vi "IV.vi"() -> ()   [LabVIEW 2018]
uses:
  Classes/2D/IV/IV.lvclass
  Classes/2D/IV/data/IV_data.lvclass
  Classes/2D/IV/meas/IV_meas.lvclass
  support/Message Queue/Enqueue Message (Single).vi
  Classes/Abstract/Measurement/Measurement2D/Measurement2D.lvclass
  Classes/Abstract/Data/Data2D/Data2D.lvclass
  support/Message Queue/Kapitza Message Queue.lvlib
  support/User Event - Stop/Kapitza User Event - Stop.lvlib
panel:
  out "Current Step":dbl[unit]
  out "dV/dI":dbl caption="dV/dI, Ohm"
  in  "Tab Control":enum32{"IV", "dV/dI (I)"}(tab)
  out "IV":cluster{"X":dbl[], "Y":dbl[]}[](graph)
  out "dV/dI (I)":cluster{"X":dbl[], "Y":dbl[]}[](graph) caption="IV"
  in  "File Path Control":path=path "C:/Users/Sergei/Documents"
  in  "Driver 1":path=path "C:/Users/Sergei/YandexDisk/Лаборатория/Projects/Kapitza_prealpha/Drivers/Simulator.vi" caption="Current source driver"
  in  "Driver 2":path=path "C:/Users/Sergei/YandexDisk/Лаборатория/Projects/Kapitza_prealpha/Drivers/Simulator.vi" caption="Voltmeter driver"
  in  "Address 2":refnum<visa-resource-name> caption="Voltmeter"
  in  "Address 1":refnum<visa-resource-name> caption="Current source"
  in  "Stop":bool
  in  "Sample Name":string
  in  "Max":dbl caption="Max current, uA"
  in  "Step":dbl caption="Current step, uA"
  in  "Init":dbl caption="Init current, uA"
  in  "x0,5 step":bool
  out "V":dbl caption="V, uV"
  out "I":dbl caption="I, uA"
  in  "x2 step":bool
  in  "Start":bool
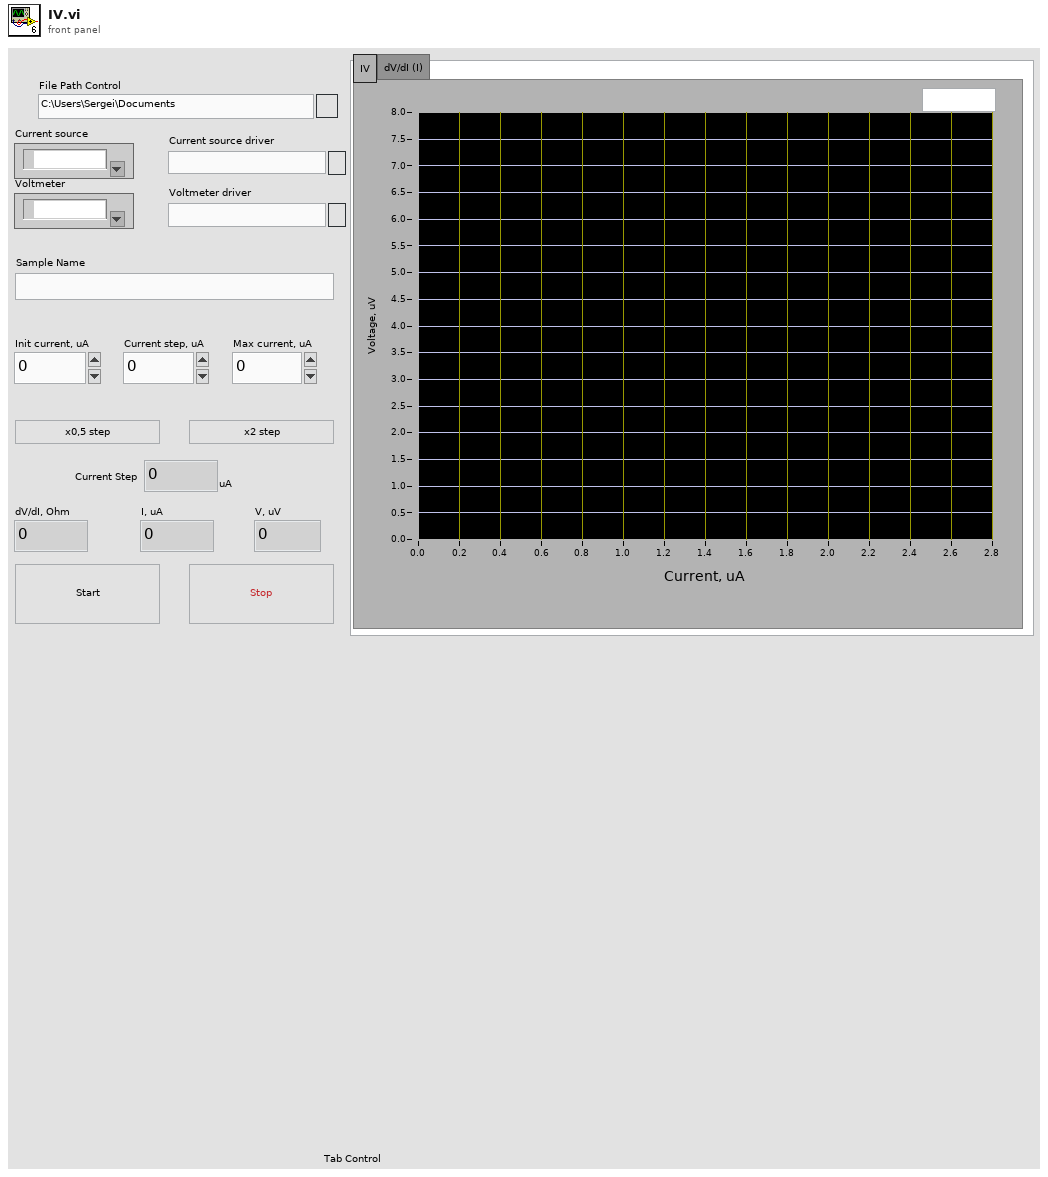
[diagram p1: front panel]
types:
  T1 = typedef "Kapitza Message Queue.lvlib/All Message Queues.ctl" = cluster{"UI":refnum<queue>}
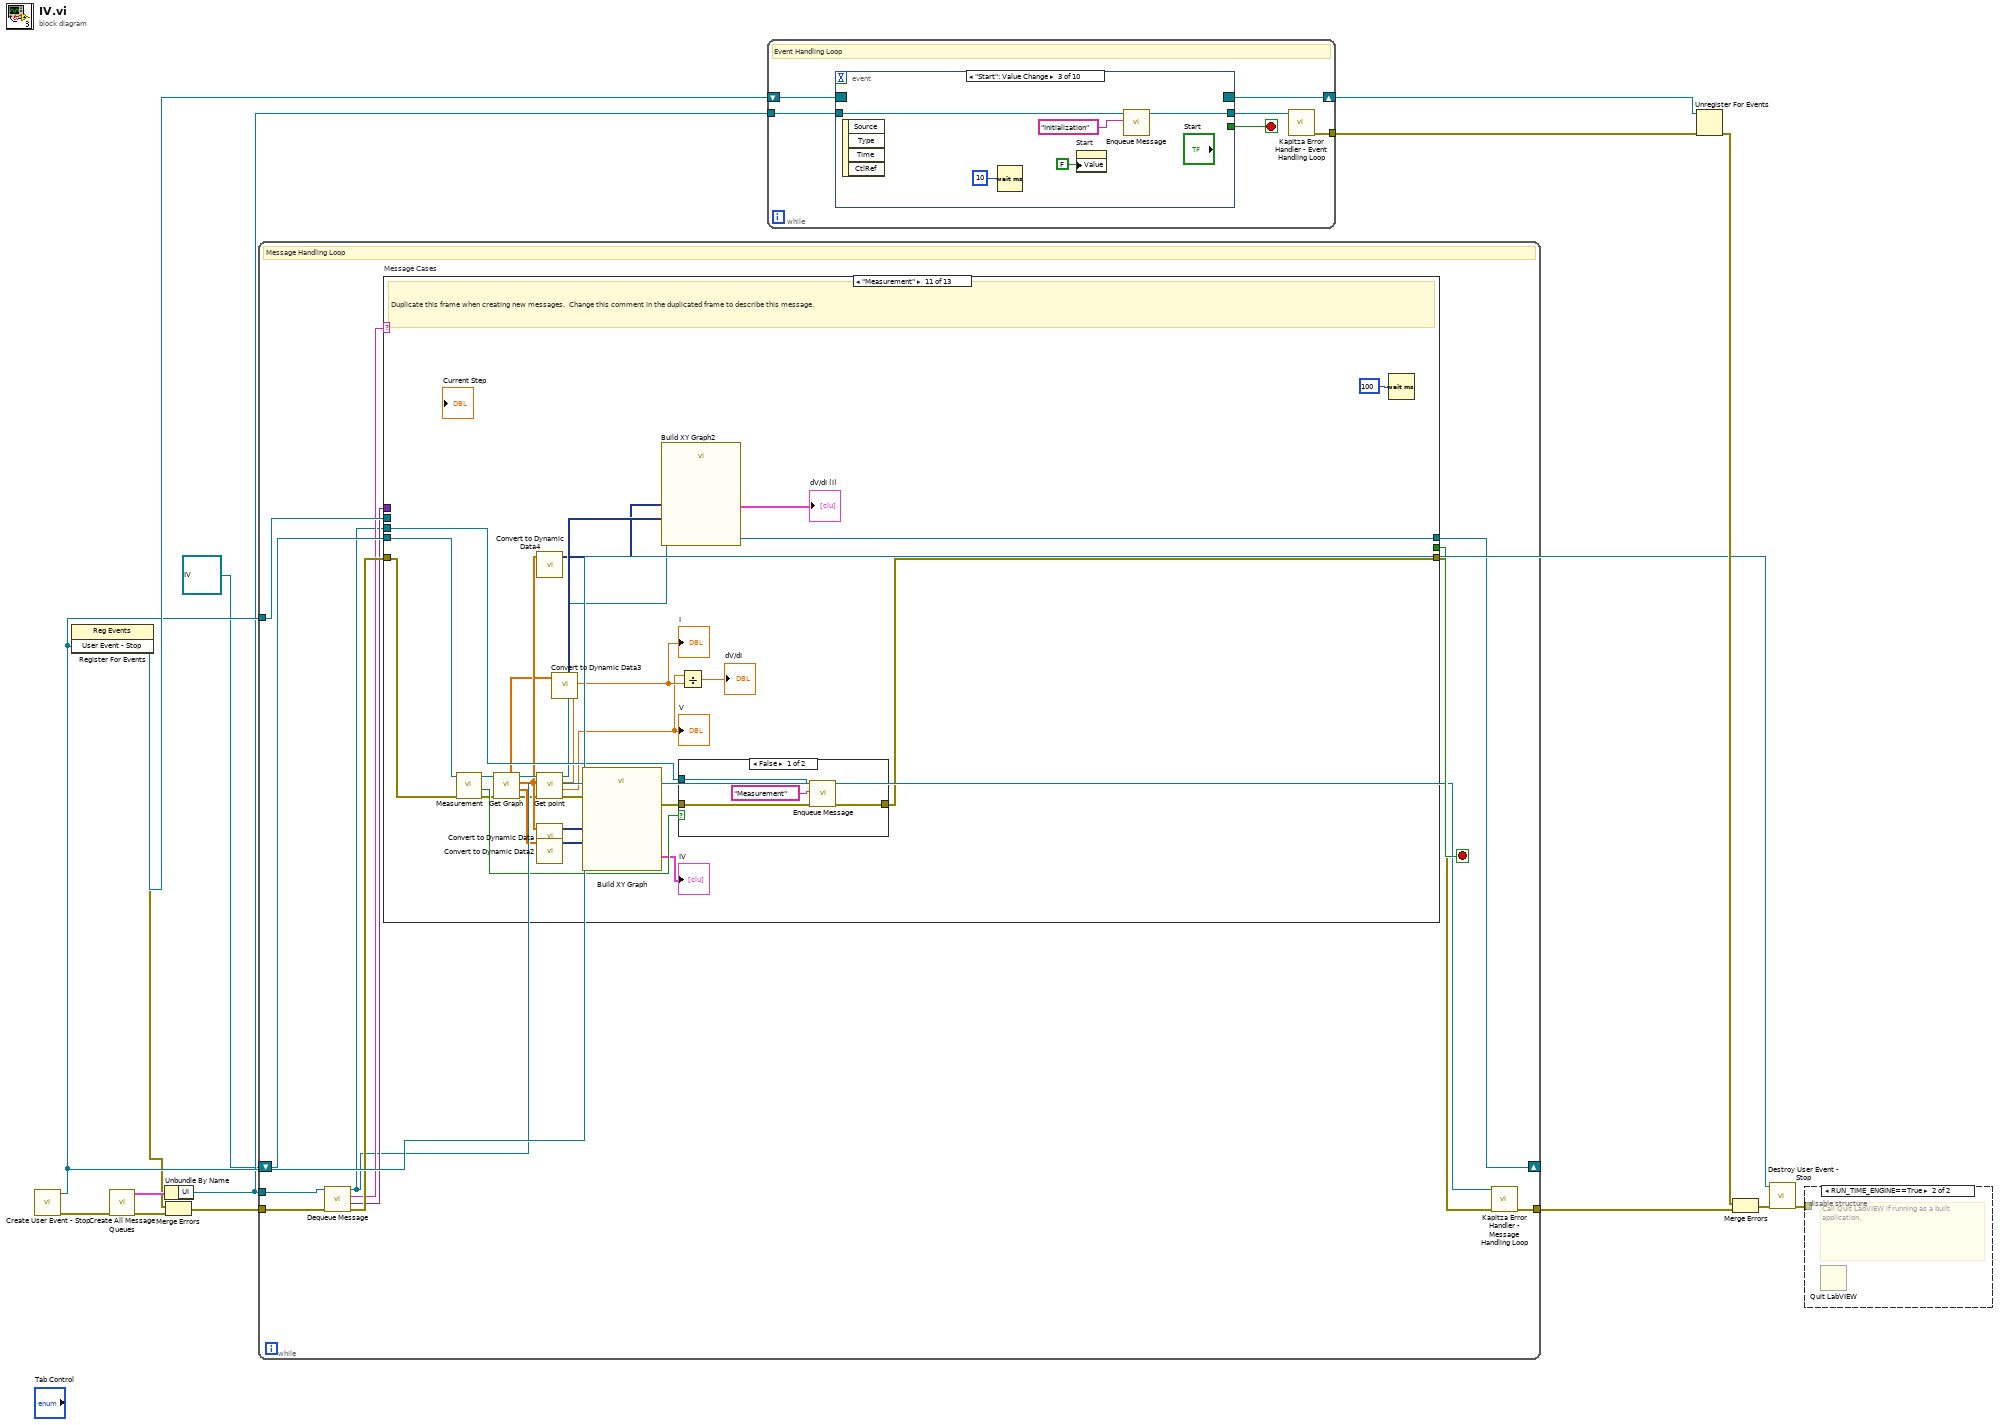
[diagram p0: block diagram]
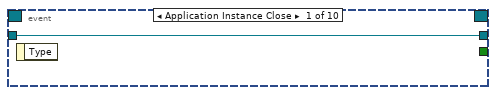
[diagram p3: hidden frame]
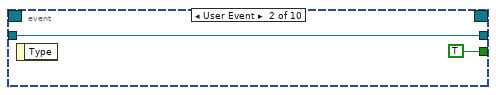
[diagram p4: hidden frame]
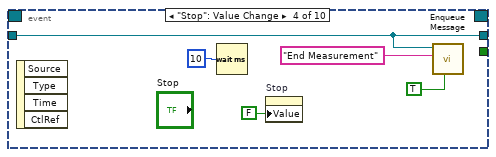
[diagram p5: hidden frame]
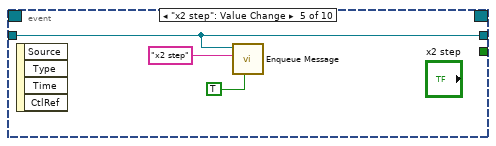
[diagram p6: hidden frame]
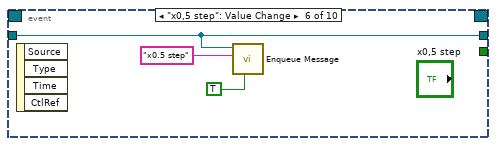
[diagram p7: hidden frame]
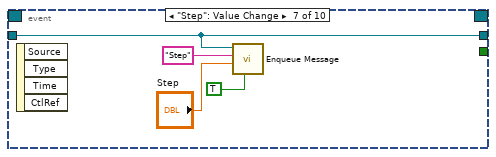
[diagram p8: hidden frame]
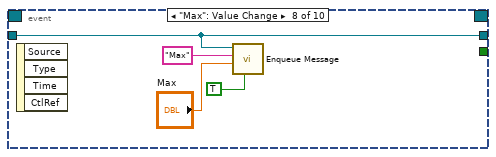
[diagram p9: hidden frame]
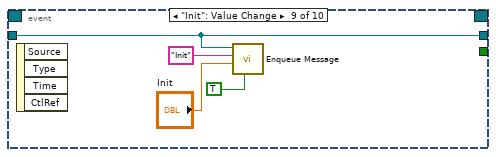
[diagram p10: hidden frame]
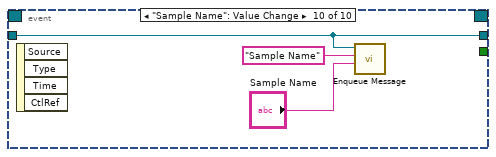
[diagram p11: hidden frame]
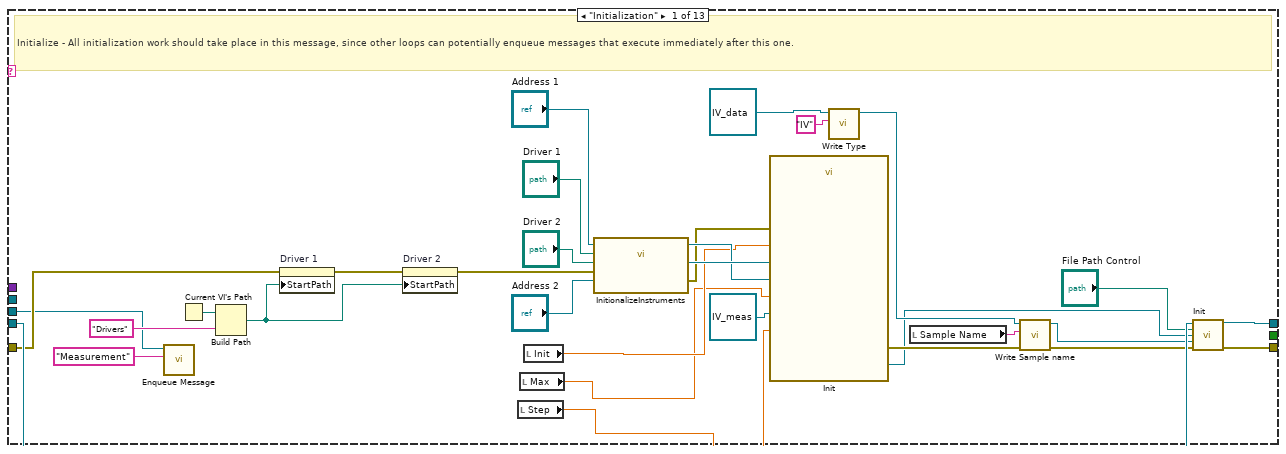
[diagram p12: hidden frame]
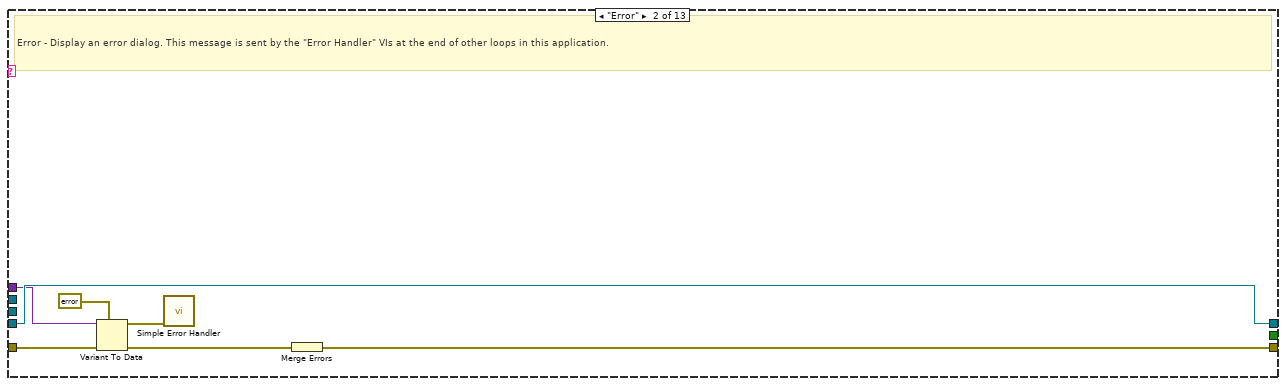
[diagram p13: hidden frame]
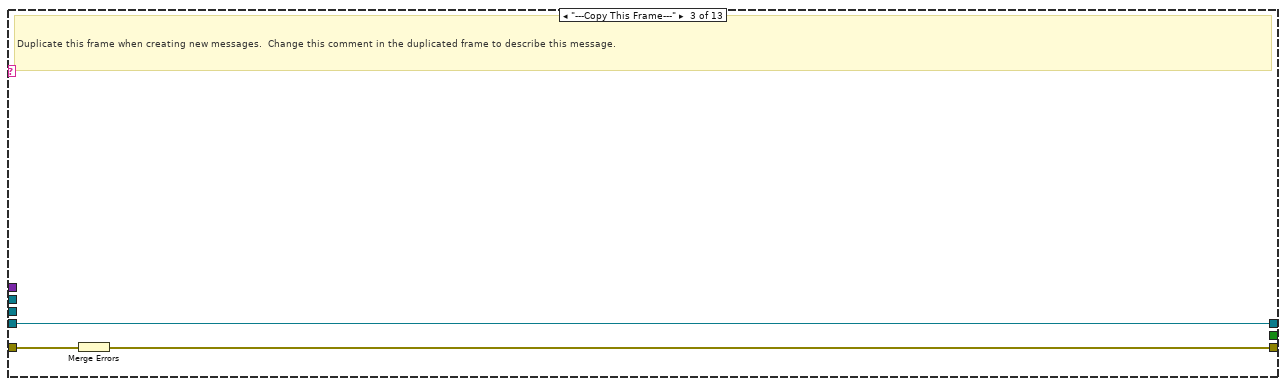
[diagram p14: hidden frame]
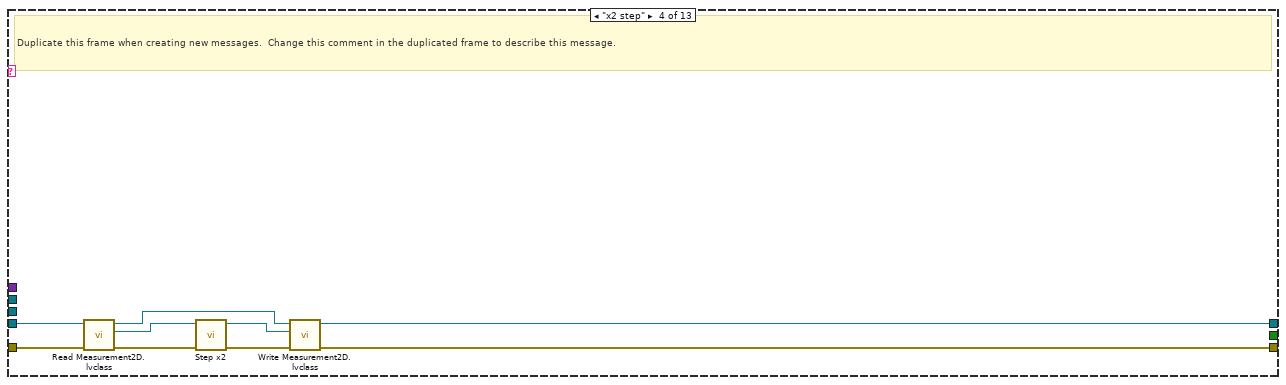
[diagram p15: hidden frame]
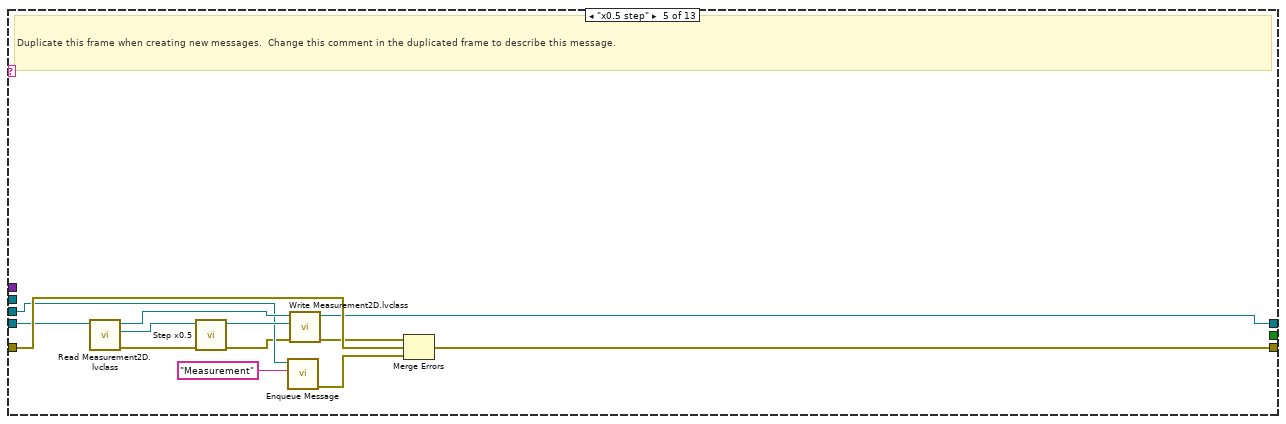
[diagram p16: hidden frame]
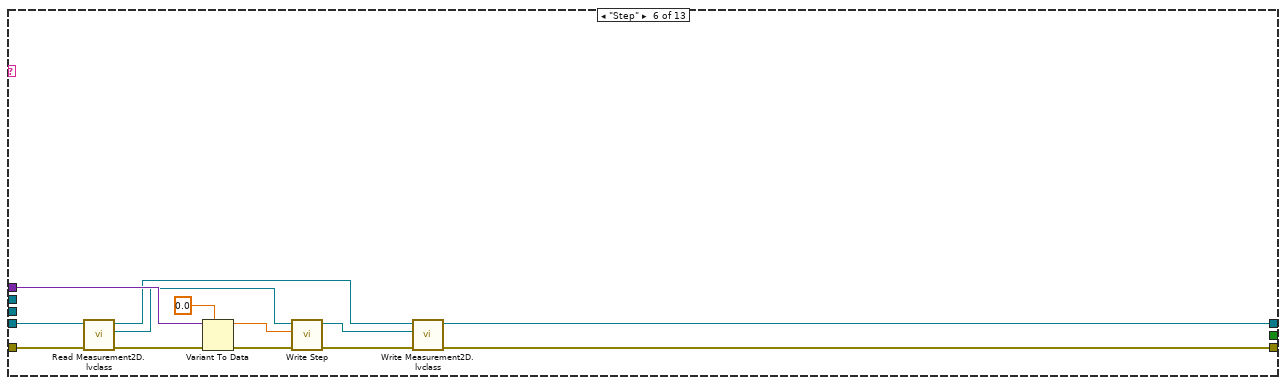
[diagram p17: hidden frame]
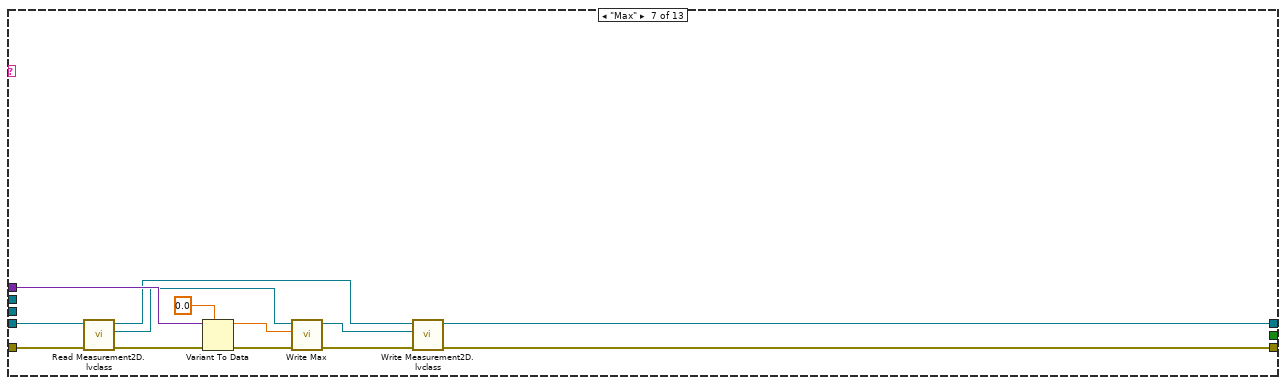
[diagram p18: hidden frame]
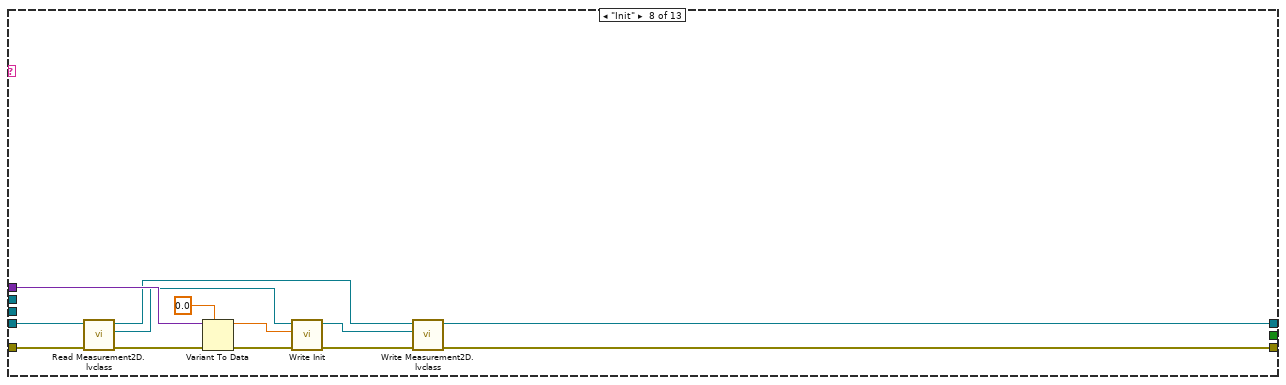
[diagram p19: hidden frame]
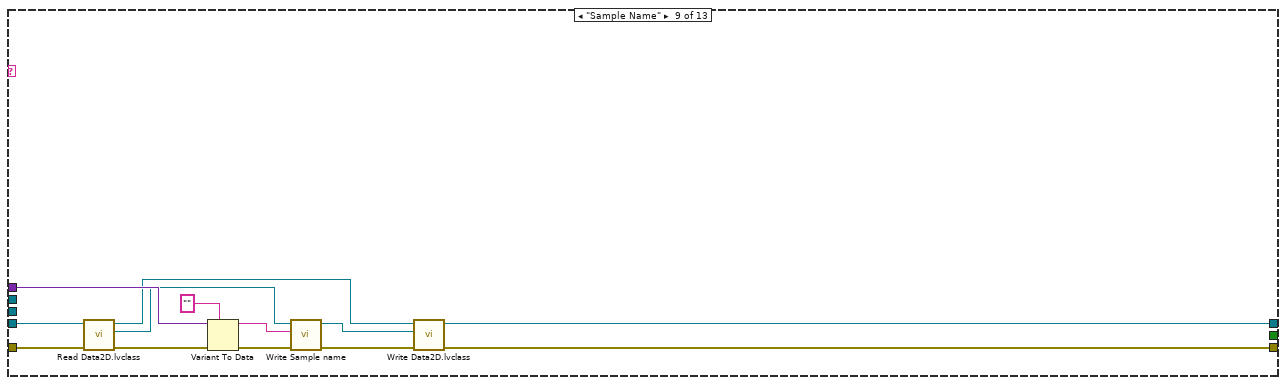
[diagram p20: hidden frame]
diagram:
  n1 = call "Create User Event - Stop.vi"() -> ("error out"=w13:errorcluster, "User Event - Stop"=w6:refnum<user-event>)  [unwired: 10 in]
  n2 = register-events(w6) -> (reference out=w7:refnum<event-registration>, error out=w4:errorcluster)  [unwired: 2 in]
  n3 = call "Create All Message Queues.vi"("error in (no error)"=w13) -> ("error out"=w2:errorcluster, "Message Queues out"=w15:T1)  [unwired: 9 in]
  n4 = Unbundle By Name(w15) -> ("UI"=w3:refnum<queue>)
  n5 = Merge Errors(w4, w2) -> (w5:errorcluster)
  n6 = while {
    tunnel: w3 -> [w19]
    shift-right: [w26] -> _
    shift-left: refnum<class "IV.lvclass"> refnum ("IV.lvclass") -> [w27]
    tunnel: w6 -> [w24]
    tunnel: w5 -> [w23]
    tunnel: [w17] -> w14
    stop <- w25 stop-if-true
    # "Message Handling Loop"
    n7 = call "Dequeue Message.vi"("error in (no error)"=w23, "Message Queue"=w19) -> ("error out"=w22:errorcluster, "Message Data"=w20:variant, "Message"=w21:string, "dup Message Queue"=w18:refnum<queue>)  [unwired: 6 in]
    n8 = case "Message Cases" shown="\"Measurement\"" w21 {
      tunnel: w18 -> [w39 _ _ _ w83 _ _ _ _ w152 w176 w197 _]
      tunnel: w22 -> [w44 w65 w68 w70 w90 w94 w108 w121 w134 w151 w170 w190 w198]
      tunnel: [w35 w59 w66 w69 w89 w91 w104 w117 w130 w149 w175 w193 w198] -> w16
      tunnel: w27 -> [w58 w64 w67 w77 w88 w100 w110 w126 w140 w153 w178 w196 w199]
      tunnel: [w57 w64 w67 w73 w86 w99 w109 w125 w139 w148 w163 w196 w199] -> w26
      tunnel: [_ _ _ _ _ _ _ _ _ _ _ TRUE _] -> w25
      tunnel: w20 -> [_ w63 _ _ _ w103 w116 w129 w142 _ _ w187 _]
      tunnel: w24 -> [_ _ _ _ _ _ _ _ _ _ _ w192 _]
      frame "Initialization" {
        # "Initialize - All initialization work should take place in this message, since other loops can potentially enqueue messages that execute immediately after this one."
        n9 = call-poly "Enqueue Message.vi"("Message"="Measurement", "Message Queue"=w39) -> ()  [unwired: 8 in, 2 out]
        n10 = Current VI's Path() -> (path=w46:path)
        n11 = Build Path(base path=w46, name or relative path="Drivers") -> (appended path=w42:path)
        n12 = property on="Driver 1" class="Path"(error in=w44, "StartPath"=w42) -> (error out=w43:errorcluster)  [unwired: 1 in, 1 out]
        n13 = property on="Driver 2" class="Path"(error in=w43, "StartPath"=w42) -> (error out=w41:errorcluster)  [unwired: 1 in, 1 out]
        n14 = local read "Step"() -> (w28:dbl)
        n15 = local read "Max"() -> (w29:dbl)
        n16 = local read "Init"() -> (w30:dbl)
        n17 = call "InitionalizeInstruments.vi"("Address in"="Address 2", "error in (no error)"=w41, "Driver in"="Driver 2", "Driver 1"="Driver 1", "VISA Refnum in"="Address 1") -> ("error out"=w49:errorcluster, "Instrument out 2"=w52:refnum<class "Instrument.lvclass">, "Instrument out"=w51:refnum<class "Instrument.lvclass">)  [unwired: 4 in]
        n18 = call-dynamic "Init.vi"("Instrument.lvclass 2"=w51, "Step"=w28, "Instrument.lvclass"=w52, "error in (no error)"=w49, "Max"=w29, "Init"=w30, "Measurement1D in"=refnum<class "IV_meas.lvclass"> refnum ("IV_meas.lvclass")) -> ("error out"=w48:errorcluster, "Measurement1D out"=w32:refnum<class "IV_meas.lvclass">)  [unwired: 3 in]
        n19 = call-dynamic "Write Type.vi"("Type"="IV", "IV_data in"=refnum<class "IV_data.lvclass"> refnum ("IV_data.lvclass")) -> ("IV_data out"=w37:refnum<class "IV_data.lvclass">)  [unwired: 8 in, 1 out]
        n20 = local read "Sample Name"() -> (w50:string)
        n21 = call-dynamic "Write Sample name.vi"("error in (no error)"=w48, "Sample name"=w50, "IV_data in"=w37) -> ("error out"=w47:errorcluster, "IV_data out"=w31:refnum<class "IV_data.lvclass">)  [unwired: 7 in]
        n22 = call-dynamic "Init.vi"("IV in"=w58, "Path"="File Path Control", "Measurement2D.lvclass"=w32, "Data2D.lvclass"=w31, "error in (no error)"=w47) -> ("IV out"=w57:refnum<class "IV.lvclass">, "error out"=w35:errorcluster)  [unwired: 9 in]
      }
      frame "Error" {
        # "Error - Display an error dialog. This message is sent by the \"Error Handler\" VIs at the end of other loops in this application."
        n23 = Variant To Data(error in=w65, type=errorcluster {"status"=FALSE, "code"=0, "source"=""} ("error constant"), Variant=w63) -> (data=w61:errorcluster, error out=w60:errorcluster)
        n24 = call <vilib>:"Simple Error Handler.vi"("error in (no error)"=w61) -> ()  [unwired: 4 in, 5 out]
        n25 = Merge Errors(w60) -> (w59:errorcluster)
      }
      frame "---Copy This Frame---" {
        # "Duplicate this frame when creating new messages.  Change this comment in the duplicated frame to describe this message."
        n26 = Merge Errors(w68) -> (w66:errorcluster)
      }
      frame "x2 step" {
        # "Duplicate this frame when creating new messages.  Change this comment in the duplicated frame to describe this message."
        n27 = call-dynamic "Read Measurement2D.lvclass.vi"("error in (no error)"=w70, "Experiment2D in"=w77) -> ("error out"=w72:errorcluster, "Measurement2D.lvclass"=w76:refnum<class "Measurement2D.lvclass">, "Experiment2D out"=w75:refnum<class "IV.lvclass">)  [unwired: 7 in]
        n28 = call-dynamic "Step x2.vi"("error in (no error)"=w72, "Measurement2D in"=w76) -> ("error out"=w71:errorcluster, "Measurement2D out"=w74:refnum<class "Measurement2D.lvclass">)  [unwired: 8 in]
        n29 = call-dynamic "Write Measurement2D.lvclass.vi"("error in (no error)"=w71, "Measurement2D.lvclass"=w74, "Experiment2D in"=w75) -> ("error out"=w69:errorcluster, "Experiment2D out"=w73:refnum<class "IV.lvclass">)  [unwired: 7 in]
      }
      frame "x0.5 step" {
        # "Duplicate this frame when creating new messages.  Change this comment in the duplicated frame to describe this message."
        n30 = call-dynamic "Read Measurement2D.lvclass.vi"("Experiment2D in"=w88) -> ("error out"=w78:errorcluster, "Measurement2D.lvclass"=w85:refnum<class "Measurement2D.lvclass">, "Experiment2D out"=w87:refnum<class "IV.lvclass">)  [unwired: 8 in]
        n31 = call-dynamic "Step x0.5.vi"("error in (no error)"=w78, "Measurement2D in"=w85) -> ("error out"=w79:errorcluster, "Measurement2D out"=w84:refnum<class "Measurement2D.lvclass">)  [unwired: 8 in]
        n32 = call-poly "Enqueue Message.vi"("Message"="Measurement", "Message Queue"=w83) -> ("error out"=w80:errorcluster)  [unwired: 8 in, 1 out]
        n33 = call-dynamic "Write Measurement2D.lvclass.vi"("error in (no error)"=w79, "Measurement2D.lvclass"=w84, "Experiment2D in"=w87) -> ("error out"=w81:errorcluster, "Experiment2D out"=w86:refnum<class "IV.lvclass">)  [unwired: 7 in]
        n34 = Merge Errors(w81, w90, w80) -> (w89:errorcluster)
      }
      frame "Step" {
        n35 = call-dynamic "Read Measurement2D.lvclass.vi"("error in (no error)"=w94, "Experiment2D in"=w100) -> ("error out"=w93:errorcluster, "Measurement2D.lvclass"=w98:refnum<class "Measurement2D.lvclass">, "Experiment2D out"=w101:refnum<class "IV.lvclass">)  [unwired: 7 in]
        n36 = Variant To Data(error in=w93, type=0.0, Variant=w103) -> (data=w97:dbl, error out=w92:errorcluster)
        n37 = call-dynamic "Write Step.vi"("error in (no error)"=w92, "Step"=w97, "Measurement2D in"=w98) -> ("error out"=w95:errorcluster, "Measurement2D out"=w96:refnum<class "Measurement2D.lvclass">)  [unwired: 7 in]
        n38 = call-dynamic "Write Measurement2D.lvclass.vi"("error in (no error)"=w95, "Measurement2D.lvclass"=w96, "Experiment2D in"=w101) -> ("error out"=w91:errorcluster, "Experiment2D out"=w99:refnum<class "IV.lvclass">)  [unwired: 7 in]
      }
      frame "Max" {
        n39 = call-dynamic "Read Measurement2D.lvclass.vi"("error in (no error)"=w108, "Experiment2D in"=w110) -> ("error out"=w107:errorcluster, "Measurement2D.lvclass"=w113:refnum<class "Measurement2D.lvclass">, "Experiment2D out"=w111:refnum<class "IV.lvclass">)  [unwired: 7 in]
        n40 = Variant To Data(error in=w107, type=0.0, Variant=w116) -> (data=w114:dbl, error out=w106:errorcluster)
        n41 = call-dynamic "Write Max.vi"("error in (no error)"=w106, "Max"=w114, "Measurement2D in"=w113) -> ("error out"=w105:errorcluster, "Measurement2D out"=w112:refnum<class "Measurement2D.lvclass">)  [unwired: 7 in]
        n42 = call-dynamic "Write Measurement2D.lvclass.vi"("error in (no error)"=w105, "Measurement2D.lvclass"=w112, "Experiment2D in"=w111) -> ("error out"=w104:errorcluster, "Experiment2D out"=w109:refnum<class "IV.lvclass">)  [unwired: 7 in]
      }
      frame "Init" {
        n43 = call-dynamic "Read Measurement2D.lvclass.vi"("error in (no error)"=w121, "Experiment2D in"=w126) -> ("error out"=w120:errorcluster, "Measurement2D.lvclass"=w124:refnum<class "Measurement2D.lvclass">, "Experiment2D out"=w127:refnum<class "IV.lvclass">)  [unwired: 7 in]
        n44 = Variant To Data(error in=w120, type=0.0, Variant=w129) -> (data=w123:dbl, error out=w119:errorcluster)
        n45 = call-dynamic "Write Init.vi"("error in (no error)"=w119, "Init"=w123, "Measurement2D in"=w124) -> ("error out"=w118:errorcluster, "Measurement2D out"=w122:refnum<class "Measurement2D.lvclass">)  [unwired: 7 in]
        n46 = call-dynamic "Write Measurement2D.lvclass.vi"("error in (no error)"=w118, "Measurement2D.lvclass"=w122, "Experiment2D in"=w127) -> ("error out"=w117:errorcluster, "Experiment2D out"=w125:refnum<class "IV.lvclass">)  [unwired: 7 in]
      }
      frame "Sample Name" {
        n47 = call-dynamic "Read Data2D.lvclass.vi"("error in (no error)"=w134, "Experiment2D in"=w140) -> ("error out"=w133:errorcluster, "Data2D.lvclass"=w137:refnum<class "Data2D.lvclass">, "Experiment2D out"=w135:refnum<class "IV.lvclass">)  [unwired: 7 in]
        n48 = Variant To Data(error in=w133, type="", Variant=w142) -> (data=w138:string, error out=w132:errorcluster)
        n49 = call-dynamic "Write Sample name.vi"("error in (no error)"=w132, "Sample name"=w138, "Data2D in"=w137) -> ("error out"=w131:errorcluster, "Data2D out"=w136:refnum<class "Data2D.lvclass">)  [unwired: 7 in]
        n50 = call-dynamic "Write Data2D.lvclass.vi"("error in (no error)"=w131, "Data2D.lvclass"=w136, "Experiment2D in"=w135) -> ("error out"=w130:errorcluster, "Experiment2D out"=w139:refnum<class "IV.lvclass">)  [unwired: 7 in]
      }
      frame "End Measurement" {
        n51 = Flush Queue(queue=w152, error in (no error)=w151) -> (error out=w150:errorcluster)  [unwired: 2 out]
        n52 = call-dynamic "End.vi"("error in (no error)"=w150, "IV in"=w153) -> ("error out"=w146:errorcluster, "IV out"=w147:refnum<class "IV.lvclass">)  [unwired: 8 in]
        n53 = call "Create Result.vi"("error in (no error)"=w146, "IV in"=w147) -> ("error out"=w143:errorcluster, "Text"=w144:string, "IV out"=w145:refnum<class "IV.lvclass">)  [unwired: 7 in]
        n54 = call-dynamic "Save.vi"("error in (no error)"=w143, "Text"=w144, "IV in"=w145) -> ("error out"=w149:errorcluster, "IV out"=w148:refnum<class "IV.lvclass">)  [unwired: 7 in]
      }
      frame "Measurement" {
        # "Duplicate this frame when creating new messages.  Change this comment in the duplicated frame to describe this message."
        n55 = call-dynamic "Measurement.vi"("error in (no error)"=w170, "IV in"=w178) -> ("error out"=w157:errorcluster, "Finish?"=w177:bool, "IV out"=w162:refnum<class "IV.lvclass">)  [unwired: 6 in, 1 out]
        n56 = call "Get Graph.vi"("error in (no error)"=w157, "IV in"=w162) -> ("error out"=w156:errorcluster, "Y"=w158:dbl[], "X"=w160:dbl[], "IV out"=w161:refnum<class "IV.lvclass">, "dY/dX"=w159:dbl[])  [unwired: 5 in]
        n57 = call "Convert to Dynamic Data4"("Array"=w160) -> ("Dynamic Data Type"=w165:dynamicdata)  [unwired: 3 in]
        n58 = call-dynamic "Get point.vi"("error in (no error)"=w156, "IV in"=w161) -> ("error out"=w171:errorcluster, "y"=w154:dbl, "x"=w155:dbl, "IV out"=w163:refnum<class "IV.lvclass">)  [unwired: 6 in]
        "I" <- w155
        "V" <- w154
        n59 = call "Convert to Dynamic Data"("Array"=w160) -> ("Dynamic Data Type"=w168:dynamicdata)  [unwired: 3 in]
        n60 = call "Convert to Dynamic Data2"("Array"=w158) -> ("Dynamic Data Type"=w173:dynamicdata)  [unwired: 3 in]
        n61 = call "Convert to Dynamic Data3"("Array"=w159) -> ("Dynamic Data Type"=w166:dynamicdata)  [unwired: 3 in]
        n62 = call "Build XY Graph"("error in (no error)"=w171, "Y Input"=w173, "X Input"=w168) -> ("error out"=w169:errorcluster, "XY Graph"=→"IV":cluster{"X":dbl[], "Y":dbl[]}[])  [unwired: 7 in]
        n63 = call "Build XY Graph2"("Y Input"=w166, "X Input"=w165) -> ("XY Graph"=→"dV/dI (I)":cluster{"X":dbl[], "Y":dbl[]}[])  [unwired: 8 in, 1 out]
        n64 = case shown="False" w177 {
          tunnel: w176 -> [w181 w186]
          tunnel: w169 -> [w180 w184]
          tunnel: [w179 w183] -> w175
          frame False {
            n65 = call-poly "Enqueue Message.vi"("error in (no error)"=w180, "Message"="Measurement", "Message Queue"=w181) -> ("error out"=w179:errorcluster)  [unwired: 7 in, 1 out]
          }
          frame True {
            n66 = call-poly "Enqueue Message.vi"("error in (no error)"=w184, "Message"="End Measurement", "Message Queue"=w186) -> ("error out"=w183:errorcluster)  [unwired: 7 in, 1 out]
          }
        }
        n67 = Divide(x=w154, y=w155) -> (x/y=→"dV/dI":dbl)
        n68 = Wait (ms)(milliseconds to wait=u32 100) -> ()  [unwired: 1 out]
      }
      frame "Exit" {
        # "Exit - Exit the application."
        n69 = Release Queue(queue=w197, error in (no error)=w190) -> (error out=w194:errorcluster)  [unwired: 1 in, 2 out]
        n70 = call "Fire User Event - Stop.vi"("User Event - Stop"=w192) -> ("error out"=w191:errorcluster)  [unwired: 10 in]
        n71 = Variant To Data(type=errorcluster {"status"=FALSE, "code"=0, "source"=""} ("error constant"), Variant=w187) -> (data=w188:errorcluster)  [unwired: 1 in, 1 out]
        n72 = call <vilib>:"Simple Error Handler.vi"("error in (no error)"=w188) -> ()  [unwired: 4 in, 5 out]
        n73 = Merge Errors(w191, w194) -> (w193:errorcluster)
      }
      frame Default {
        # "'Default' case only runs if there is a message that isn't defined in any of the other cases"
      }
    }
    n74 = call "Kapitza Error Handler - Message Handling Loop.vi"("error in (no error)"=w16, "Message Queue"=w18) -> ("dup error in"=w17:errorcluster)  [unwired: 8 in, 1 out]
  }
  n75 = while {
    tunnel: w3 -> [w205]
    shift-right: [w203] -> w10
    shift-left: w7 -> [w204]
    tunnel: [w200] -> w8
    stop <- w202 stop-if-true
    # "Event Handling Loop"
    n76 = event shown="[2] \"Start\": Value Change" {
      selector: w204 -> [_ _ _ _ _ _ _ _ _ _]
      dyn-events: [_ _ _ _ _ _ _ _ _ _] -> w203
      timeout: _ -> [_ _ _ _ _ _ _ _ _ _]
      tunnel: [_ TRUE ("Discard?") _ _ _ _ _ _ _ _] -> w202
      tunnel: w205 -> [w206 w208 w213 w218 w221 w222 w227 w230 w234 w238]
      tunnel: [w206 w208 w212 w218 w221 w222 w227 w230 w234 w238] -> w201
      event Application Instance Close {
        n77 = event-data() -> ()  [unwired: 1 in, 1 out]
      }
      event User Event {
        n78 = event-data() -> ()  [unwired: 1 in, 1 out]
      }
      event "Start": Value Change {
        n79 = event-data() -> ()  [unwired: 1 in, 4 out]
        n80 = Wait (ms)(milliseconds to wait=u32 10) -> ()  [unwired: 1 out]
        n81 = property on="Start" class="Bool (strict)"("Value"=FALSE ("Start")) -> ()  [unwired: 2 in, 2 out]
        n82 = call-poly "Enqueue Message.vi"("Message"="Initialization", "Message Queue"=w213) -> ("dup Message Queue"=w212:refnum<queue>)  [unwired: 8 in, 1 out]
      }
      event "Stop": Value Change {
        n83 = event-data() -> ()  [unwired: 1 in, 4 out]
        n84 = Wait (ms)(milliseconds to wait=u32 10) -> ()  [unwired: 1 out]
        n85 = property on="Stop" class="Bool (strict)"("Value"=FALSE ("Stop")) -> ()  [unwired: 2 in, 2 out]
        n86 = call-poly "Enqueue Message.vi"("Priority Message? (F)"=TRUE, "Message"="End Measurement", "Message Queue"=w218) -> ()  [unwired: 7 in, 2 out]
      }
      event "x2 step": Value Change {
        n87 = event-data() -> ()  [unwired: 1 in, 4 out]
        n88 = call-poly "Enqueue Message.vi"("Priority Message? (F)"=TRUE, "Message"="x2 step", "Message Queue"=w221) -> ()  [unwired: 7 in, 2 out]
      }
      event "x0,5 step": Value Change {
        n89 = event-data() -> ()  [unwired: 1 in, 4 out]
        n90 = call-poly "Enqueue Message.vi"("Priority Message? (F)"=TRUE, "Message"="x0.5 step", "Message Queue"=w222) -> ()  [unwired: 7 in, 2 out]
      }
      event "Step": Value Change {
        n91 = event-data() -> ()  [unwired: 1 in, 4 out]
        n92 = call-poly "Enqueue Message.vi"("Priority Message? (F)"=TRUE, "Message Data"="Step", "Message"="Step", "Message Queue"=w227) -> ()  [unwired: 6 in, 2 out]
      }
      event "Max": Value Change {
        n93 = event-data() -> ()  [unwired: 1 in, 4 out]
        n94 = call-poly "Enqueue Message.vi"("Priority Message? (F)"=TRUE, "Message Data"="Max", "Message"="Max", "Message Queue"=w230) -> ()  [unwired: 6 in, 2 out]
      }
      event "Init": Value Change {
        n95 = event-data() -> ()  [unwired: 1 in, 4 out]
        n96 = call-poly "Enqueue Message.vi"("Priority Message? (F)"=TRUE, "Message Data"="Init", "Message"="Init", "Message Queue"=w234) -> ()  [unwired: 6 in, 2 out]
      }
      event "Sample Name": Value Change {
        n97 = event-data() -> ()  [unwired: 1 in, 4 out]
        n98 = call-poly "Enqueue Message.vi"("Message Data"="Sample Name", "Message"="Sample Name", "Message Queue"=w238) -> ()  [unwired: 7 in, 2 out]
      }
    }
    n99 = call "Kapitza Error Handler - Event Handling Loop.vi"("Message Queue"=w201) -> ("dup error in"=w200:errorcluster)  [unwired: 9 in, 1 out]
  }
  n100 = Unregister For Events(event registration refnum=w10, error in=w8) -> (error out=w11:errorcluster)
  n101 = Merge Errors(w11, w14) -> (w12:errorcluster)
  n102 = call "Destroy User Event - Stop.vi"("error in (no error)"=w12, "User Event - Stop"=w6) -> ("error out"=w9:errorcluster)  [unwired: 9 in]
  n103 = disable-structure shown="RUN_TIME_ENGINE==True" {
    disable-tunnel: w9 -> [_ _]
    frame condition #0 (active) {
    }
    frame condition #1 {
      # "Call Quit LabVIEW if running as a built application."
      n104 = Quit LabVIEW() -> ()  [unwired: 1 in]
    }
  }
